vi "JKI_Python_Server Example 2 Nodes 1 Registration.vi"() -> ()   [LabVIEW 2013]
uses:
  CallHandler/PyObject.lvclass
  Server/Register for Events (Object Array).vi
  <userlib>/_OpenG.lib/lvdata/lvdata.llb/Get Strings from Enum__ogtk.vi
  Server/Server.lvclass
  Call/Call.lvclass
panel:
  out "Number of Connections":u32
  out "Client Connected":bool
  out "error out":errorcluster
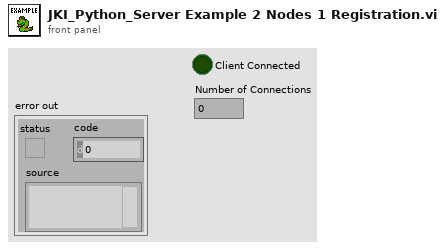
[diagram p1: front panel]
types:
  T1 = typedef "JKI_Python_Bridge_for_LV.lvlib/Server.lvclass/Python Method Call - Event Registration.ctl" = refnum<event-registration>
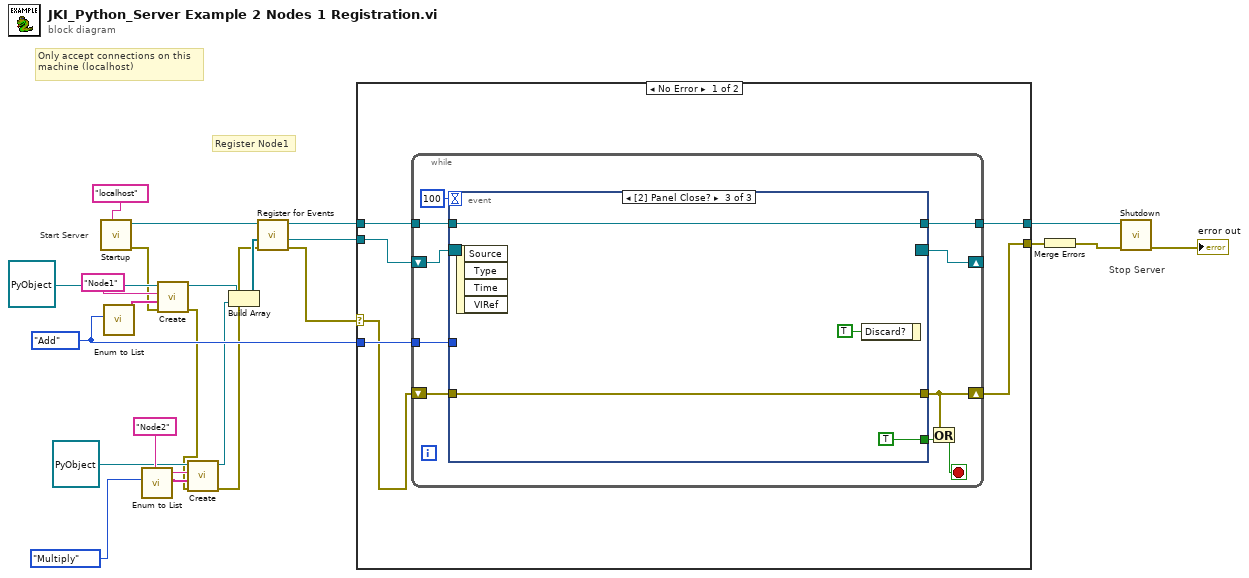
[diagram p0: block diagram]
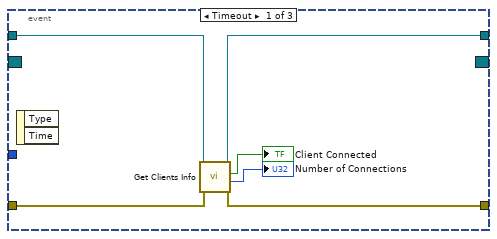
[diagram p2: hidden frame]
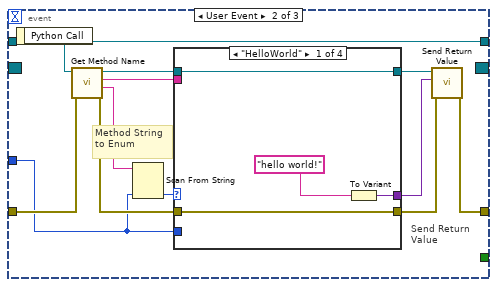
[diagram p3: hidden frame]
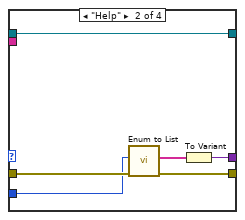
[diagram p4: hidden frame]
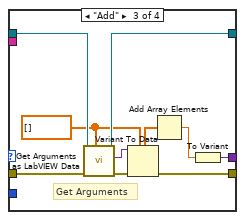
[diagram p5: hidden frame]
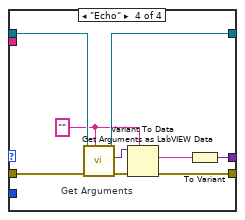
[diagram p6: hidden frame]
diagram:
  w18 = enum16{"HelloWorld", "Echo", "Add", "Help"}."Add"
  # "Register Node1"
  # "Stop Server"
  # "Start Server"
  # "Only accept connections on this machine (localhost)"
  n1 = call "Startup.vi"("IP Address (localhost)"="localhost" ("name")) -> ("error out"=w6:errorcluster, "JKI_Python_Server out"=w22:refnum<class "Server.lvclass">)  [unwired: 9 in]
  n2 = call "Enum to List.vi"("Enum"=w18) -> ("Enum Strings"=w14:string[])  [unwired: 9 in, 1 out]
  n3 = call "Enum to List.vi"("Enum"=enum16{"HelloWorld", "Echo", "Multiply", "Help"}."Multiply") -> ("Enum Strings"=w13:string[])  [unwired: 9 in, 1 out]
  n4 = call "Create.vi"("error in (no error)"=w6, "Method Names"=w14, "Object Name"="Node1" ("Python Node Name"), "Node in"=refnum<class "PyObject.lvclass"> refnum) -> ("error out"=w5:errorcluster, "Node out"=w11:refnum<class "PyObject.lvclass">)  [unwired: 6 in]
  n5 = call "Create.vi"("error in (no error)"=w5, "Method Names"=w13, "Object Name"="Node2" ("Python Node Name"), "Node in"=refnum<class "PyObject.lvclass"> refnum) -> ("error out"=w4:errorcluster, "Node out"=w9:refnum<class "PyObject.lvclass">)  [unwired: 6 in]
  n6 = Build Array(w11, w9) -> (w10:refnum<class "PyObject.lvclass">[])
  n7 = call-poly "Register for Events.vi"("error in (no error)"=w4, "PyObject []"=w10, "JKI_Python_Server in"=w22) -> ("error out"=w1:errorcluster, "Python Event"=w16:T1, "JKI_Python_Server out"=w3:refnum<class "Server.lvclass">)  [unwired: 6 in]
  n8 = case shown="No Error" w1 {
    selector: w1 -> [w24 w93]
    tunnel: [w29 w93] -> w19
    tunnel: w18 -> [w28 _]
    tunnel: w16 -> [w27 _]
    tunnel: w3 -> [w26 w92]
    tunnel: [w25 w92] -> w2
    frame No Error {
      n9 = while {
        shift-right: [w35] -> w29
        shift-left: w24 -> [w38]
        shift-right: [w36] -> _
        shift-left: w27 -> [w39]
        tunnel: w28 -> [w32]
        tunnel: w26 -> [w31]
        tunnel: [w30] -> w25
        stop <- w34 stop-if-true
        n10 = event shown="[2] Panel Close?" {
          selector: w39 -> [_ _ _]
          dyn-events: [_ _ _] -> w36
          timeout: 100 -> [_ _ _]
          tunnel: [w42 w51 w91] -> w35
          tunnel: w38 -> [w43 w56 w91]
          tunnel: [_ _ TRUE] -> w33
          tunnel: w32 -> [_ w53 _]
          tunnel: w31 -> [w41 w46 w88]
          tunnel: [w40 w46 w88] -> w30
          event Timeout {
            n11 = event-data() -> ()  [unwired: 1 in, 2 out]
            n12 = call "Get Clients Info.vi"("error in (no error)"=w43, "JKI_Python_Server in"=w41) -> ("error out"=w42:errorcluster, "Number of Connections"=→"Number of Connections":u32, "Client Connected"=→"Client Connected":bool, "JKI_Python_Server out"=w40:refnum<class "Server.lvclass">)  [unwired: 5 in, 1 out]
          }
          event User Event {
            # "Send Return\nValue"
            # "Method String to Enum"
            n13 = event-data() -> ("Python Call"=w57:refnum<class "Call.lvclass">)  [unwired: 1 in]
            n14 = call "Get Method Name.vi"("error in (no error)"=w56, "Call in"=w57) -> ("error out"=w55:errorcluster, "Method Name"=w48:string, "Object Name"=w47:string, "Call out"=w54:refnum<class "Call.lvclass">)  [unwired: 6 in]
            n15 = Scan From String(input string=w48, default 1=w53) -> (output 1=w58:enum16{"HelloWorld", "Echo", "Add", "Help"})  [unwired: 3 in, 3 out]
            n16 = case shown="\"HelloWorld\"" w58 {
              tunnel: [w59 w67 w69 w79] -> w50
              tunnel: w55 -> [w61 w66 w72 w83]
              tunnel: [w61 w65 w77 w87] -> w52
              tunnel: [w60 w68 w74 w85] -> w49
              tunnel: w54 -> [w60 w68 w75 w86]
              tunnel: w53 -> [_ w64 _ _]
              tunnel: w47 -> [_ _ _ _]
              frame "HelloWorld" {
                n17 = To Variant(anything="hello world!" ("Arguments")) -> (Variant=w59:variant)
              }
              frame "Help" {
                n18 = call "Enum to List.vi"("error in (no error)"=w66, "Enum"=w64) -> ("error out"=w65:errorcluster, "Enum Strings"=w63:string[])  [unwired: 8 in]
                n19 = To Variant(anything=w63) -> (Variant=w67:variant)
              }
              frame "Add" {
                w70 = dbl[] []
                # "Get Arguments"
                n20 = call "Get Arguments as LabVIEW Data.vi"("type"=w70, "error in (no error)"=w72, "Call in"=w75) -> ("error out"=w71:errorcluster, "LabVIEW Data"=w73:variant, "Call out"=w74:refnum<class "Call.lvclass">)  [unwired: 6 in]
                n21 = Variant To Data(error in=w71, type=w70, Variant=w73) -> (data=w78:dbl[], error out=w77:errorcluster)
                n22 = Add Array Elements(numeric array=w78) -> (sum=w76:dbl)
                n23 = To Variant(anything=w76) -> (Variant=w69:variant)
              }
              frame "Echo" {
                w81 = ""
                # "Get Arguments"
                n24 = call "Get Arguments as LabVIEW Data.vi"("type"=w81, "error in (no error)"=w83, "Call in"=w86) -> ("error out"=w82:errorcluster, "LabVIEW Data"=w84:variant, "Call out"=w85:refnum<class "Call.lvclass">)  [unwired: 6 in]
                n25 = Variant To Data(error in=w82, type=w81, Variant=w84) -> (data=w80:string, error out=w87:errorcluster)
                n26 = To Variant(anything=w80) -> (Variant=w79:variant)
              }
            }
            n27 = call "Send Return Value.vi"("error in (no error)"=w52, "Return Value"=w50, "Response in"=w49) -> ("error out"=w51:errorcluster)  [unwired: 8 in]
          }
          event Panel Close? {
            n28 = event-data() -> ()  [unwired: 1 in, 4 out]
            n29 = event-data("Discard?"=TRUE) -> ()  [unwired: 1 in, 1 out]
          }
        }
        n30 = Or(x=w35, y=w33) -> (x .or. y?=w34:bool)
      }
    }
    frame Error {
    }
  }
  n31 = Merge Errors(w19) -> (w20:errorcluster)
  n32 = call "Shutdown.vi"("error in (no error)"=w20, "JKI_Python_Server in"=w2) -> ("error out"=→"error out":errorcluster)  [unwired: 9 in]
